vi "Play Youtube Video.vi"(8 "error in (no error)":errorcluster, 10 "Youtube URL":string, 11 "VLC Wrapper in":refnum<class "VLC Wrapper.lvclass">) -> (0 "error out":errorcluster, 3 "VLC Wrapper out":refnum<class "VLC Wrapper.lvclass">)   [LabVIEW 2020, in "VLC Wrapper.lvclass"]
uses:
  VLC Wrapper.lvclass
  C:/Users/fflores/Documents/GitHub Projects/LabVIEW-CLI-Wrapper/Console Wrapper/Console Wrapper.lvclass
  Console Wrapper/Console Wrapper.lvclass/Console Wrapper.ctl
  Console Wrapper/Write Command Options.vi
  Console Wrapper/Write Command.vi
  Console Wrapper/Console Wrapper.lvclass
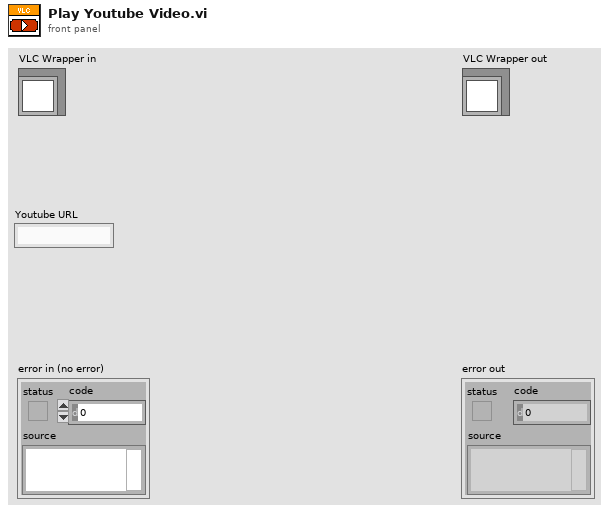
[diagram p1: front panel]
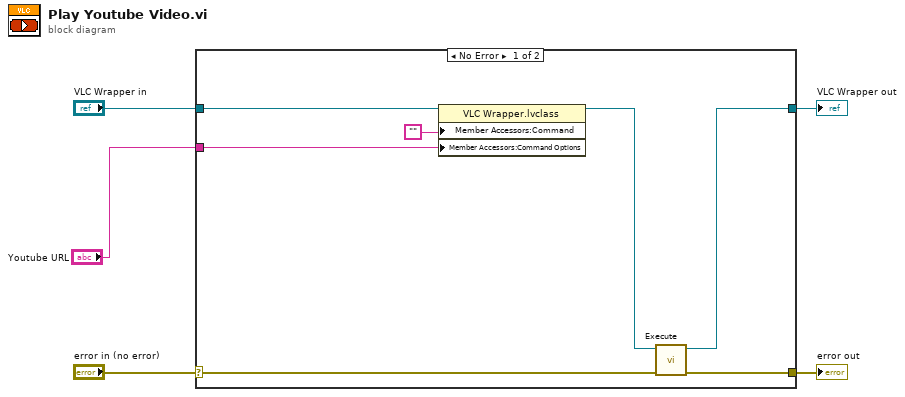
[diagram p0: block diagram]
diagram:
  n1 = case shown="No Error" "error in (no error)" {
    selector: "error in (no error)" -> [w12 w14]
    tunnel: [w11 w14] -> w4
    tunnel: [w9 w13] -> w2
    tunnel: "VLC Wrapper in" -> [w10 w13]
    tunnel: "Youtube URL" -> [w6 _]
    frame No Error {
      n2 = property class="VLC Wrapper.lvclass"(reference=w10, "Member Accessors:Command"="", "Member Accessors:Command Options"=w6) -> (reference out=w8:refnum<class "VLC Wrapper.lvclass">)  [unwired: 1 in, 1 out]
      n3 = call "Execute.vi"("error in (no error)"=w12, "Console Wrapper in"=w8) -> ("error out"=w11:errorcluster, "Console Wrapper out"=w9:refnum<class "VLC Wrapper.lvclass">)  [unwired: 7 in, 1 out]
    }
    frame Error {
    }
  }
  "error out" <- w4
  "VLC Wrapper out" <- w2
